vi "Parse MAVLink Message.vi"(11 "Instance Details":T2) -> ()   [LabVIEW 2014]
uses:
  Ground Station to Aircraft Coms/SubVI/Aircraft Data Router/Controls/Known Aircraft.ctl
  Ground Station to Aircraft Coms/SubVI/Hardware Driver/Controls/Coms Driver Interface.ctl
  Telemetry/Controls/Telemetry Connection Type.ctl
  <vilib>/httpClient/ClientHandle.ctl
  Controls/MAVLink Command ACK.ctl
  Aircraft Information/Controls/Drone Information.ctl
  Aircraft Information/Controls/Base Mode.ctl
  Aircraft Information/Controls/Aircraft Mode.ctl
  Aircraft Information/Controls/Aircraft Extra Data.ctl
  Controls/MAVLink Optical Flow.ctl
  Controls/MAVLink EKF Status Report.ctl
  Aircraft Information/Controls/Aircraft Sensor Status Data.ctl
  GUI Design/Indicators/Sensor Status LED CLuster.ctl
  GUI Design/Indicators/Status LED.ctl
  Aircraft Information/Controls/Aircraft GPS Data.ctl
  Aircraft Information/Controls/GPS Fix Type.ctl
  Aircraft Information/Controls/Aircraft Attitude Data.ctl
  Controls/MAVLink Recieved Param.ctl
  Aircraft Information/Sub VI/Set Aircraft System Status.vi
  Aircraft Information/Sub VI/Set Aircraft Information.vi
  Aircraft Information/Sub VI/Set Aircraft Extra Data.vi
  Aircraft Information/Sub VI/Set Aircraft GPS.vi
  Aircraft Information/Sub VI/Set Aircraft Attitude.vi
  Application Support/Stop Button/SubVI/Get Stop Button Status.vi
  <vilib>/httpClient/LabVIEWHTTPClient.lvlib
panel:
  out "output cluster":T1
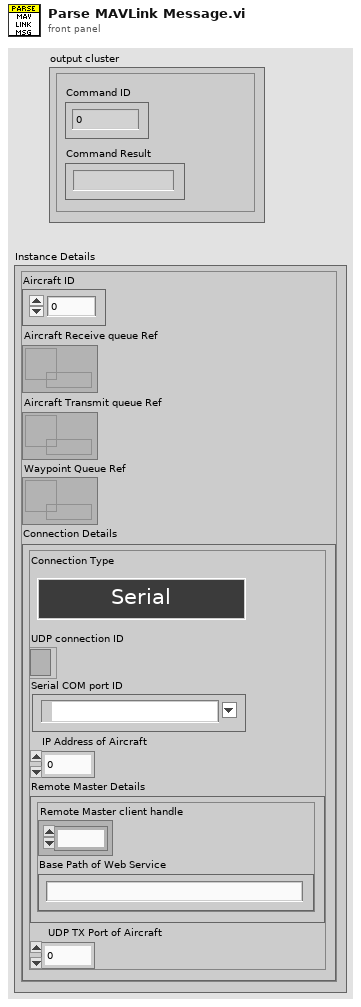
[diagram p1: front panel]
types:
  T1 = typedef "MAVLink Command ACK.ctl" = cluster{"Command ID":u16, "Command Result":string}
  T2 = typedef "Known Aircraft.ctl" = cluster{"Aircraft ID":u8, "Aircraft Receive queue Ref":refnum<queue>, "Aircraft Transmit queue Ref":refnum<queue>, "Waypoint Queue Ref":refnum<queue>, "Connection Details":T3}
  T3 = typedef "Coms Driver Interface.ctl" = cluster{"Connection Type":T4, "UDP connection ID":refnum<k16>, "Serial COM port ID":refnum<visa-resource-name>, "IP Address of Aircraft":u32, "Remote Master Details":cluster{"Remote Master client handle":T5, "Base Path of Web Service":string}, "UDP TX Port of Aircraft":u16}
  T4 = typedef "Telemetry Connection Type.ctl" = enum16{"Serial", "UDP", "Remote Master"}
  T5 = typedef "LabVIEWHTTPClient.lvlib/ClientHandle.ctl" = refnum<k1>
  T6 = typedef "Aircraft Attitude Data.ctl" = cluster{"Roll":sgl, "Pitch":sgl, "Yaw":sgl, "Timestamp":u32, "Update Frequency":dbl, "Altitude":sgl}
  T7 = typedef "Aircraft GPS Data.ctl" = cluster{"Latitude (degrees)":dbl, "Longitude (degrees)":dbl, "Altitude (m)":dbl, "Fix Type":T8, "HDOP (cm)":u16, "VDOP (cm)":u16, "Ground Speed (m/s)":dbl, "Coarse Over Ground (degrees)":u16, "Number of Satellites":u8}
  T8 = typedef "GPS Fix Type.ctl" = enum16{"No Fix 0", "No Fix 1", "2D Fix", "3D Fix", "DGPS", "RTK"}
  T9 = typedef "Aircraft Sensor Status Data.ctl" = cluster{"Sensor Status":T10, "CPU Load (%)":dbl, "Battery Voltage (V)":dbl, "Battery Current (A)":dbl, "Battery Remaining (%)":dbl, "Communication Drop Rate (%)":dbl, "Communication Errors (%)":dbl, "Status text":string}
  T10 = typedef "Sensor Status LED CLuster.ctl" = cluster{"3D Gyro":u32, "3D Accel":u32, "3D Mag":u32, "Abs. Pressure":u32, "Diff. Pressure":u32, "GPS":T11, "Optical Flow":u32, "Vision Position":u32, "Laser Position":u32, "External Ground Truth":u32, "Angular Rate Control":u32, "Attitude Stabilisation":u32, "Yaw Position":u32, "Z Altitude Control":u32, "XY Position Control":u32, "Motor Outputs":u32, "RC Receiver":u32, "3D Gyro 2":u32, "3D Accel 2":u32, "3D Mag 2":u32, "Geofence":u32, "AHRS":u32, "Terrain":u32}
  T11 = typedef "Status LED.ctl" = u32
  T12 = typedef "Aircraft Extra Data.ctl" = cluster{"Optical Flow":T13, "RNGFND Distance (m)":sgl, "RNGFND Voltage":sgl, "EKF Status Report":T14}
  T13 = typedef "MAVLink Optical Flow.ctl" = cluster{"Time (usec)":u64, "Flow Comp mx":sgl, "Flow Comp my":sgl, "Ground Distance (m)":sgl, "Flow x":i16, "Flow y":i16, "Sensord ID":u8, "Quality":u8}
  T14 = typedef "MAVLink EKF Status Report.ctl" = cluster{"EKF Status Flags":cluster{"Attitude Estimate":bool, "Horizontal Velocity":bool, "Vertical Velocity":bool, "Horizontal POS Relative":bool, "Horizontal POS Absolute":bool, "Vertical POS Relative":bool, "Vertical POS Absolute":bool, "Vertical POS AGL":bool, "Contstant POS Mode":bool, "Predicted Horizontal POS Relative":bool, "Predicted Horizontal POS Absolute":bool}, "Velocity Variance":sgl, "Horizontal POS Variance":sgl, "Vertical POS Variance":sgl, "Compass Variance":sgl, "Terrain Altitude Variance":sgl}
  T15 = typedef "Drone Information.ctl" = cluster{"Aircraft ID":u8, "Tag ID":string, "System Status":string, "Base Mode":T16, "Armed/Disarmed":bool, "Battery Voltage":dbl, "Control Mode":T17, "Initialisation":u8, "Coms with aircraft good":bool, "Mode":string, "Mission Uploaded":bool}
  T16 = typedef "Base Mode.ctl" = cluster{"Custom Mode":bool, "Test Enabled":bool, "Autonomous Mode":bool, "Guided Mode":bool, "Stabilization Enabled":bool, "HIL Enabled":bool, "Manual Mode":bool, "Arm":bool}
  T17 = typedef "Aircraft Mode.ctl" = enum16{"Loiter", "Stabalise", "Failsafe", "Emergency Stop"}
  T18 = typedef "MAVLink Recieved Param.ctl" = cluster{"Param ID":string, "Param Value":sgl, "Param Type":u8, "Param Count":u16, "Param Index":u16}
  T19 = enum16{"ALL", "RAW_SENSORS", "EXTENDED_STATUS", "RC_CHANNELS", "RAW_CONTROLLER", "POSITION", "EXTRA1", "EXTRA2", "EXTRA3"}
  T20 = cluster{"x acc":i16, "y acc":i16, "z acc":i16, "x gyro":i16, "y gyro":i16, "z gyro":i16, "x mag":i16, "y mag":i16, "z mag":i16}
  T21 = cluster{"Channel 1":u16, "Channel 2":u16, "Channel 3":u16, "Channel 4":u16, "Channel 5":u16, "Channel 6":u16, "Channel 7":u16, "Channel 8":u16}
  T22 = typedef "MAVLink Packet.ctl" = cluster{"Payload Length":u8, "Packet Sequence":u8, "System ID":u8, "Component ID":u8, "Message ID":u8, "Data":string, "Checksum":u16}
  T23 = typedef "MAVLink Heartbeat.ctl" = cluster{"custom_mode":u32, "Type":u8, "autopilot":u8, "base_mode":u8, "system_status":u8, "mavlink_version":u8, "heartbeat":bool}
  T24 = typedef "MAVLink System Status.ctl" = cluster{"onboard_control_sesnors_present":u32, "onboard_control_sesnors_enabled":u32, "onboard_control_sesnors_health":u32, "load (%*10)":u16, "voltage_battery (mV)":u16, "current_battery (mA*10)":i16, "drop_rate_comm (%*100)":u16, "error_comm":u16, "error_count1":u16, "error_count2":u16, "error_count3":u16, "error_count4":u16, "battery_remaining (%)":i8}
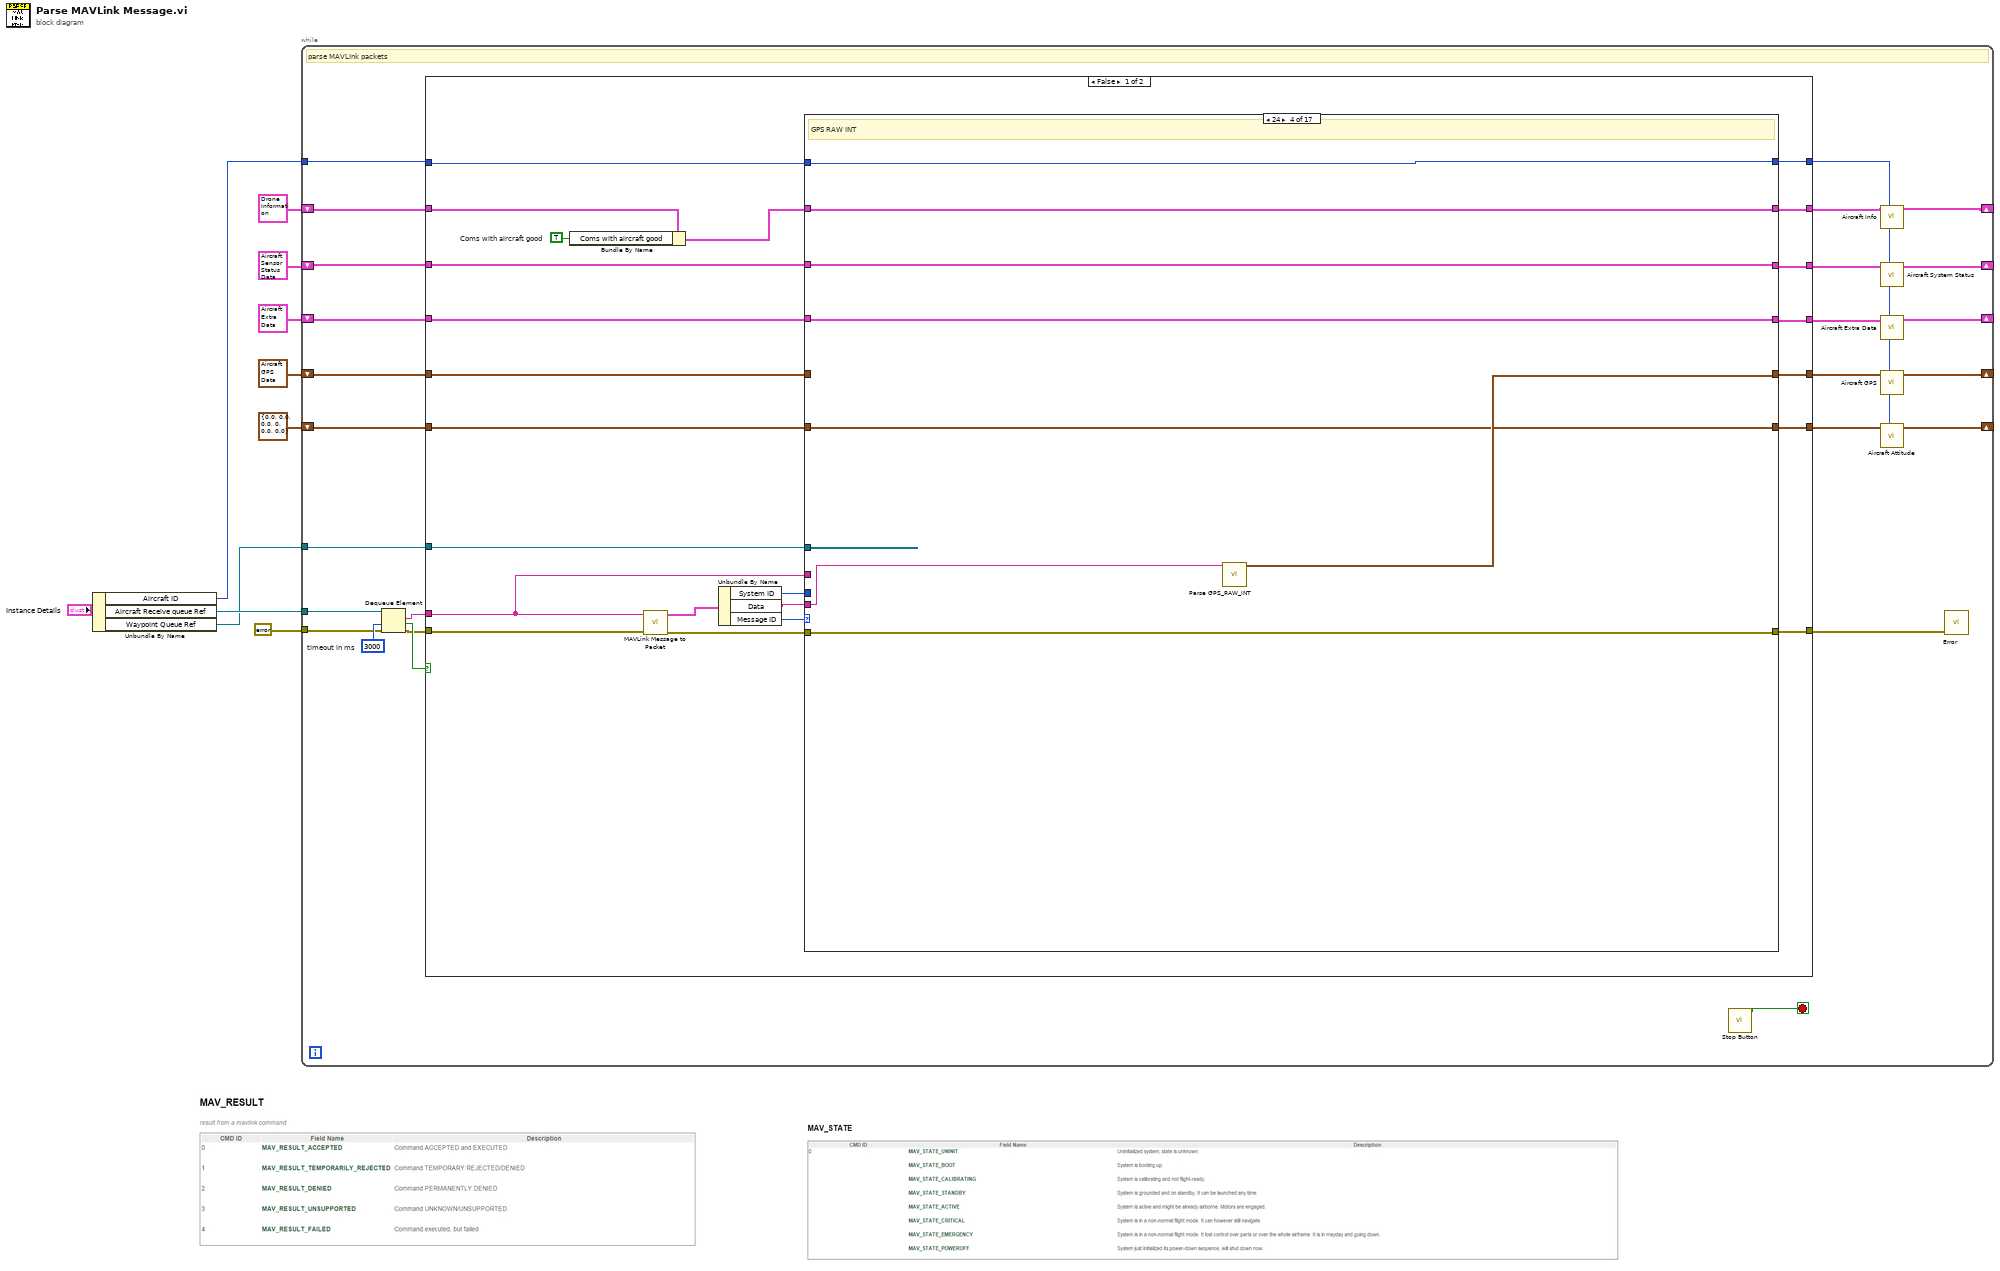
[diagram p0: block diagram]
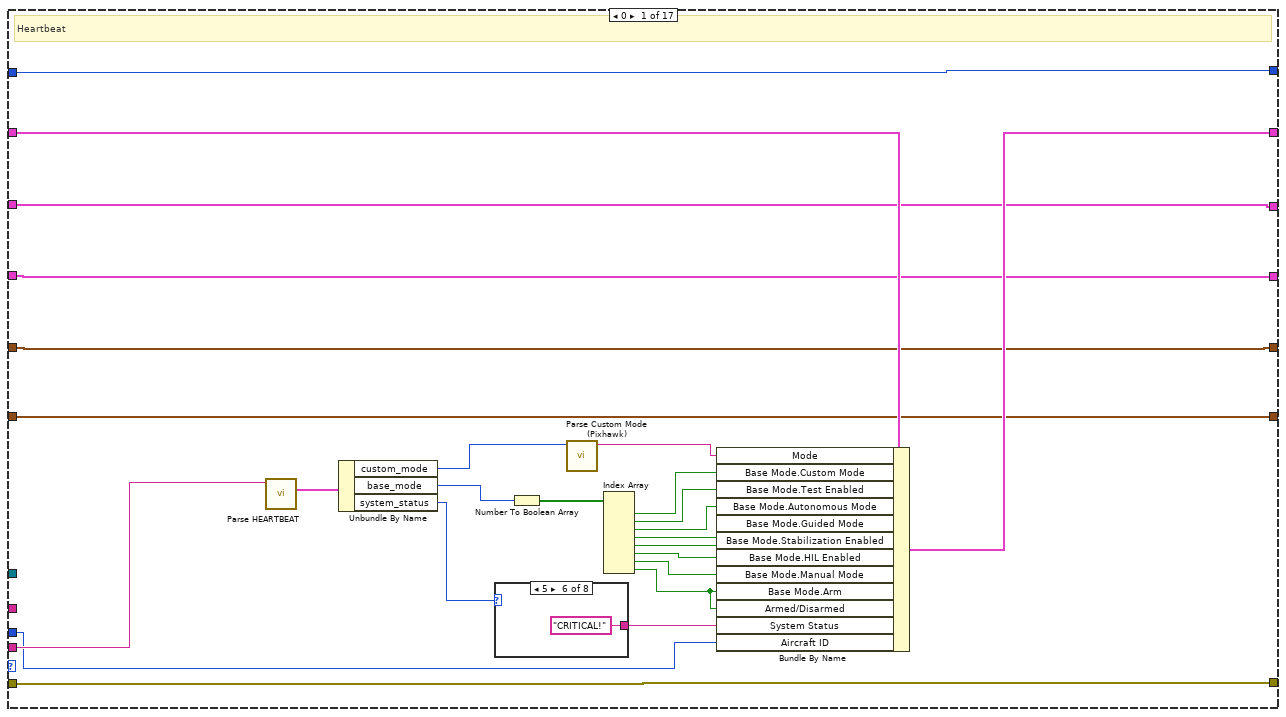
[diagram p2: hidden frame]
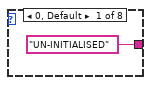
[diagram p3: hidden frame]
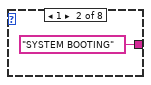
[diagram p4: hidden frame]
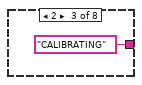
[diagram p5: hidden frame]
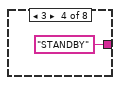
[diagram p6: hidden frame]
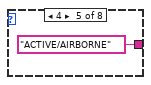
[diagram p7: hidden frame]
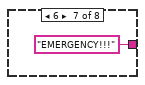
[diagram p8: hidden frame]
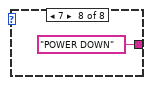
[diagram p9: hidden frame]
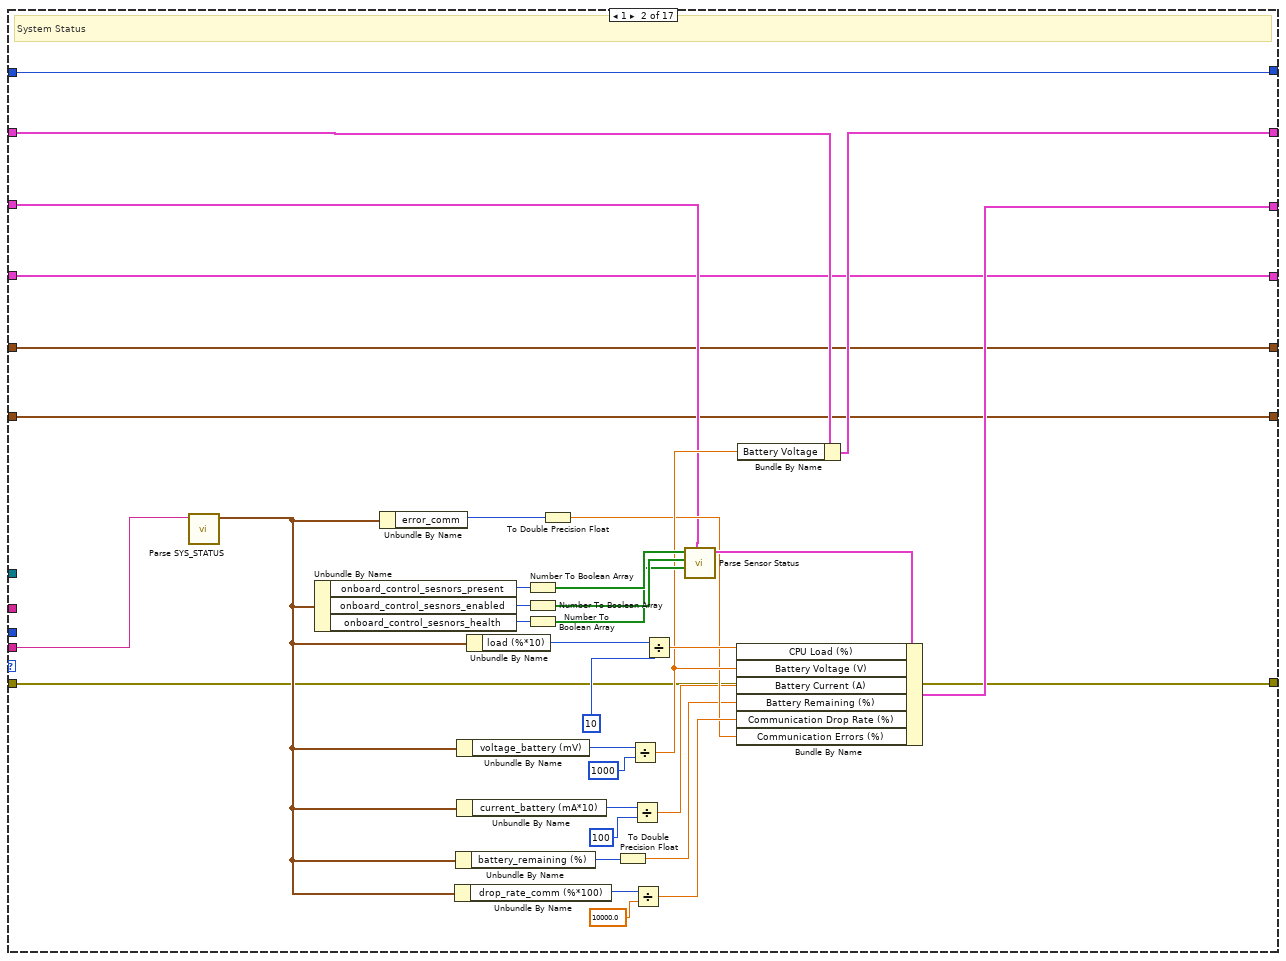
[diagram p10: hidden frame]
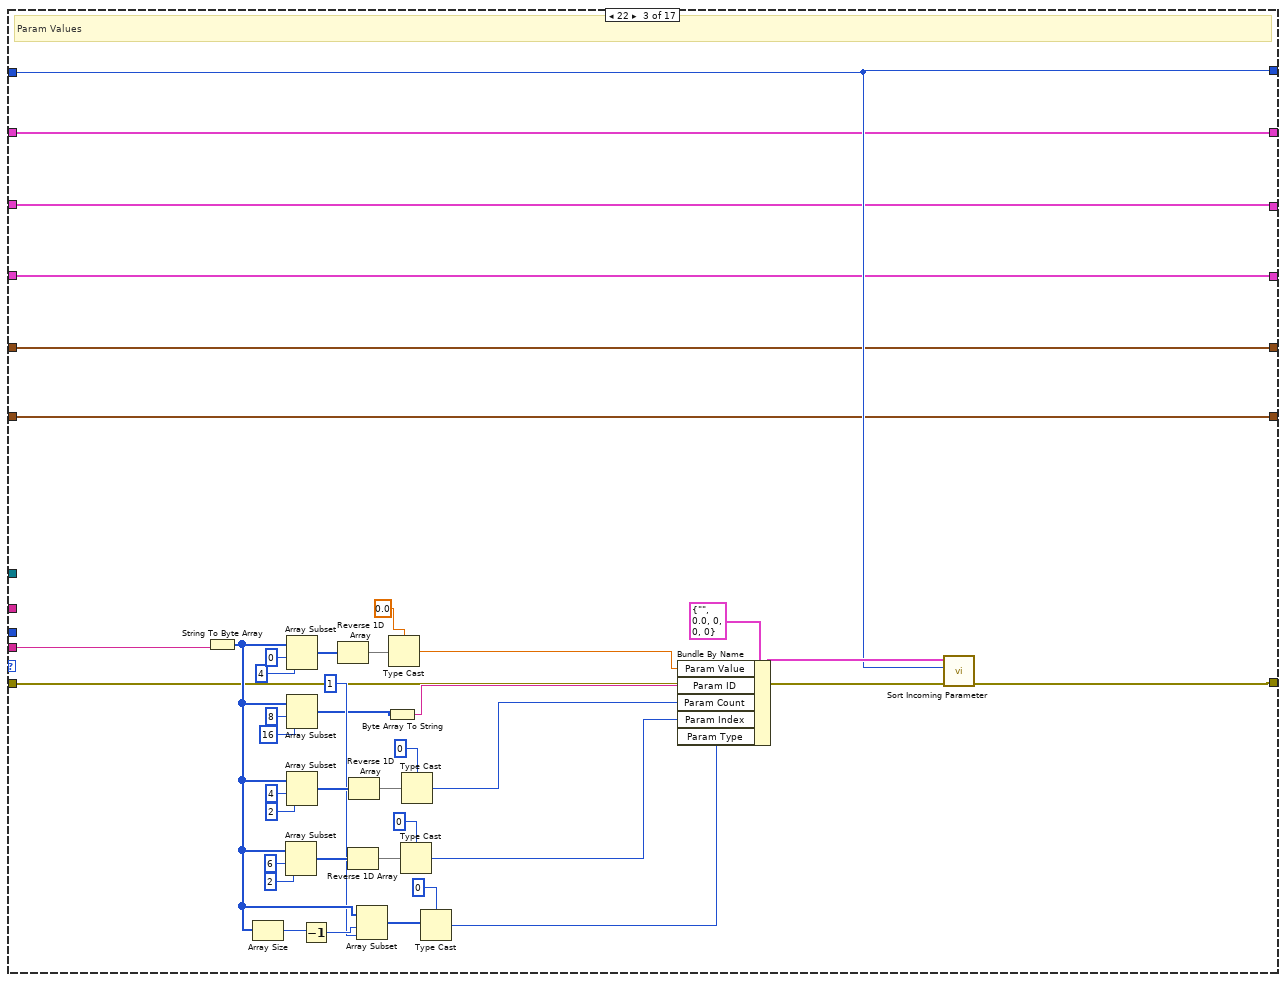
[diagram p11: hidden frame]
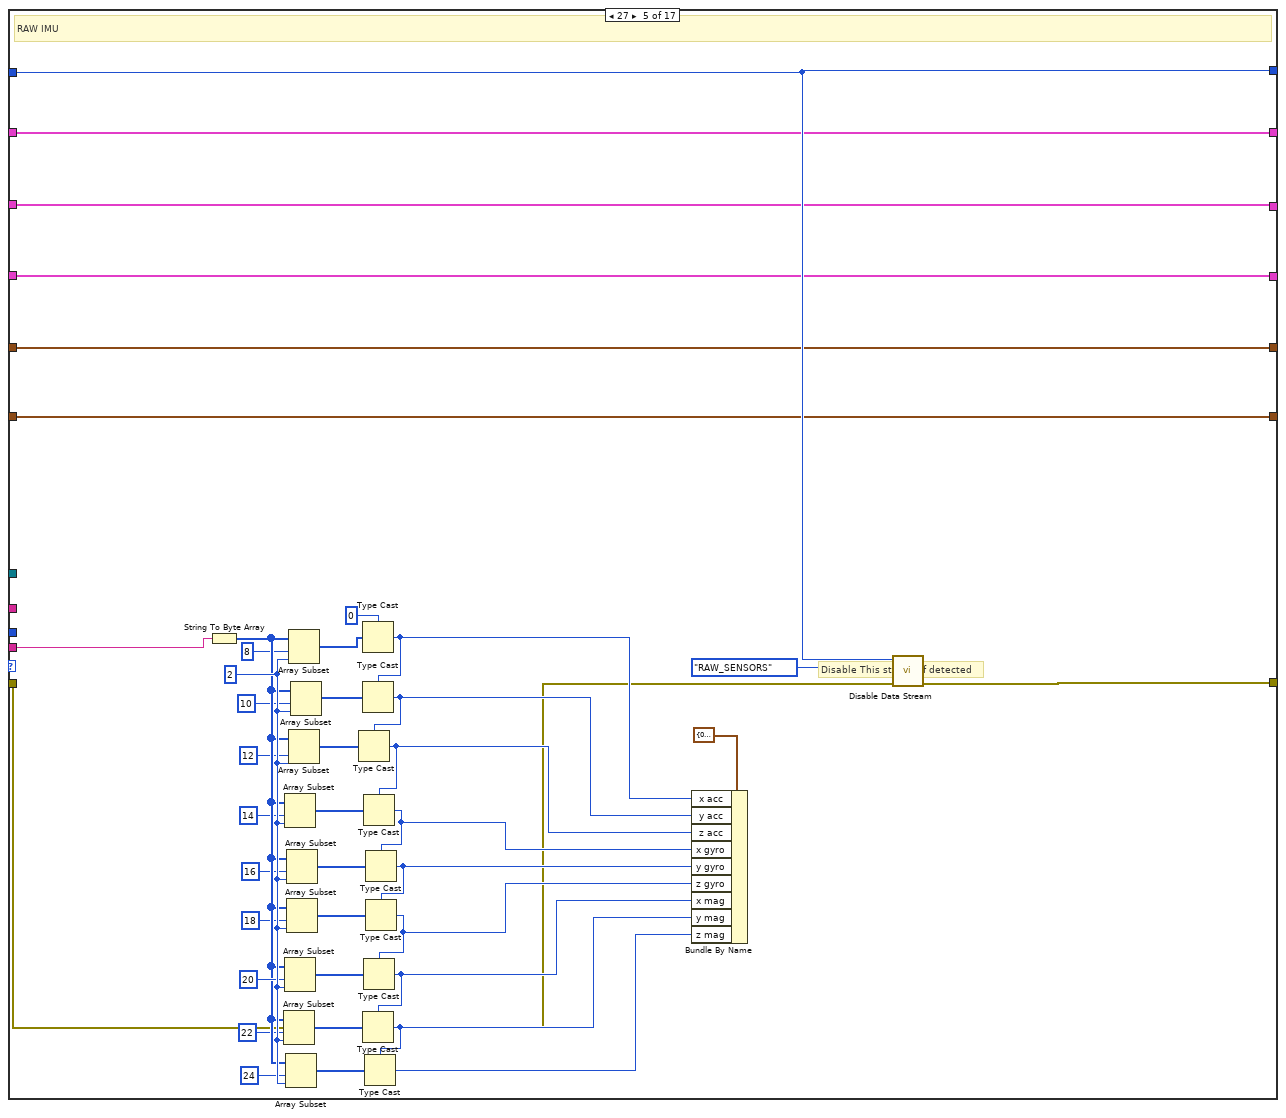
[diagram p12: hidden frame]
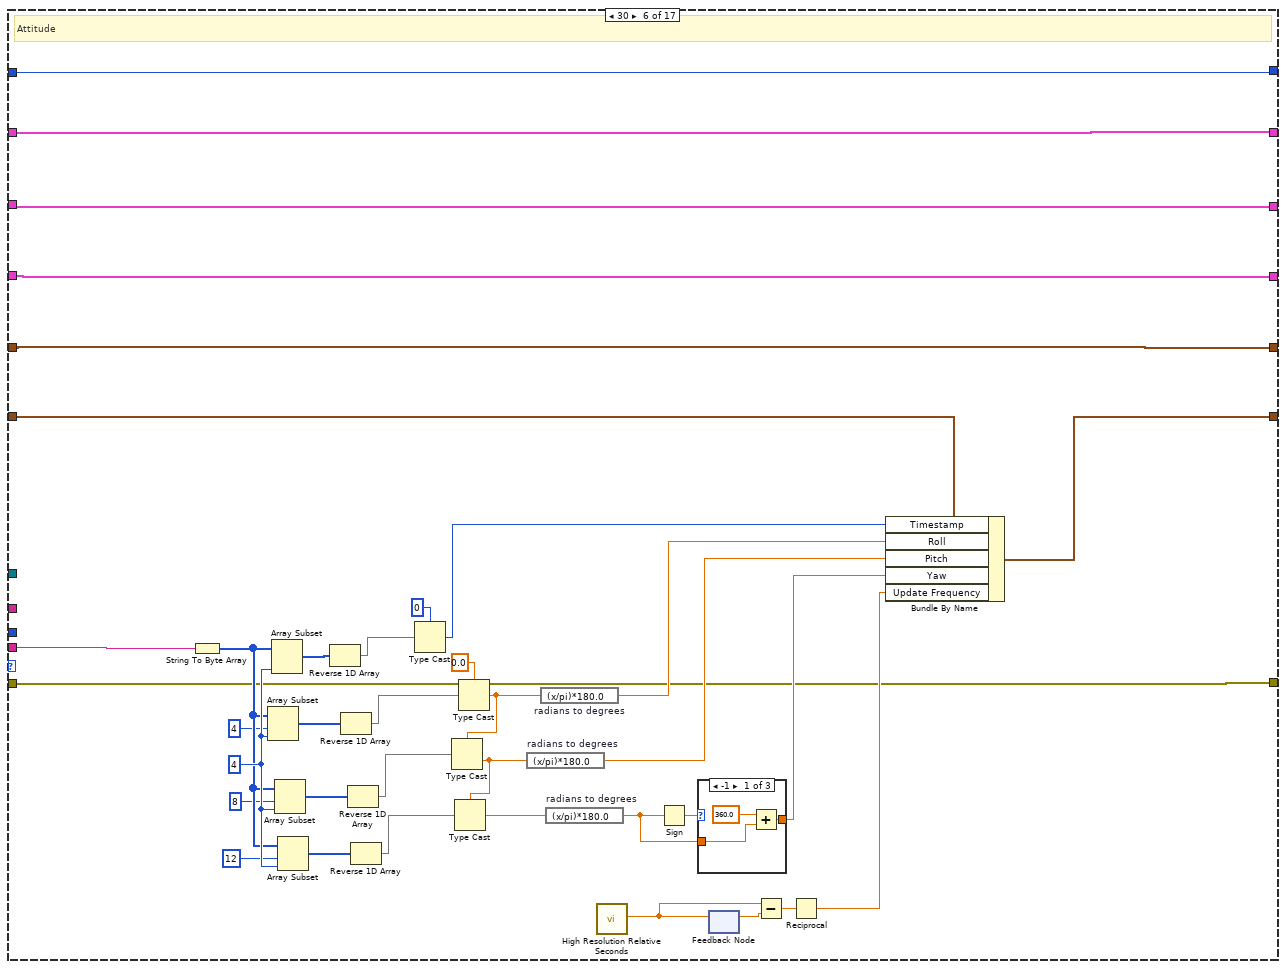
[diagram p13: hidden frame]
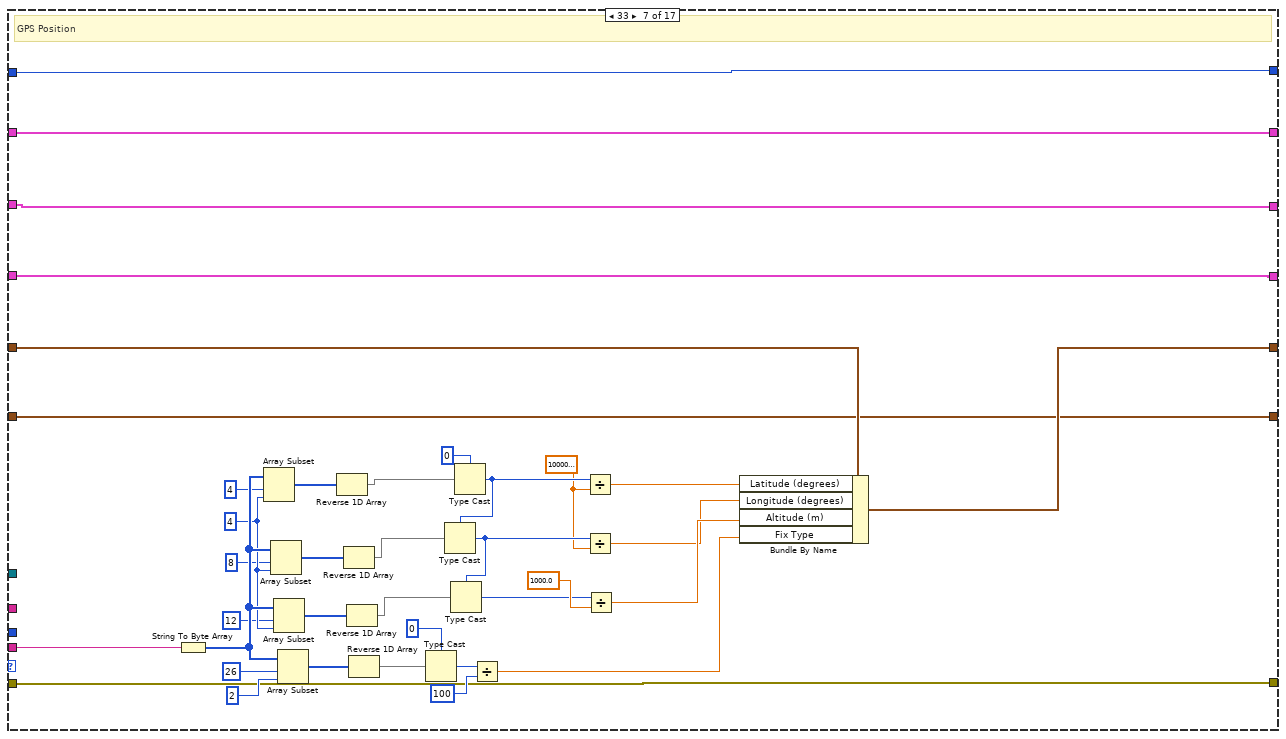
[diagram p16: hidden frame]
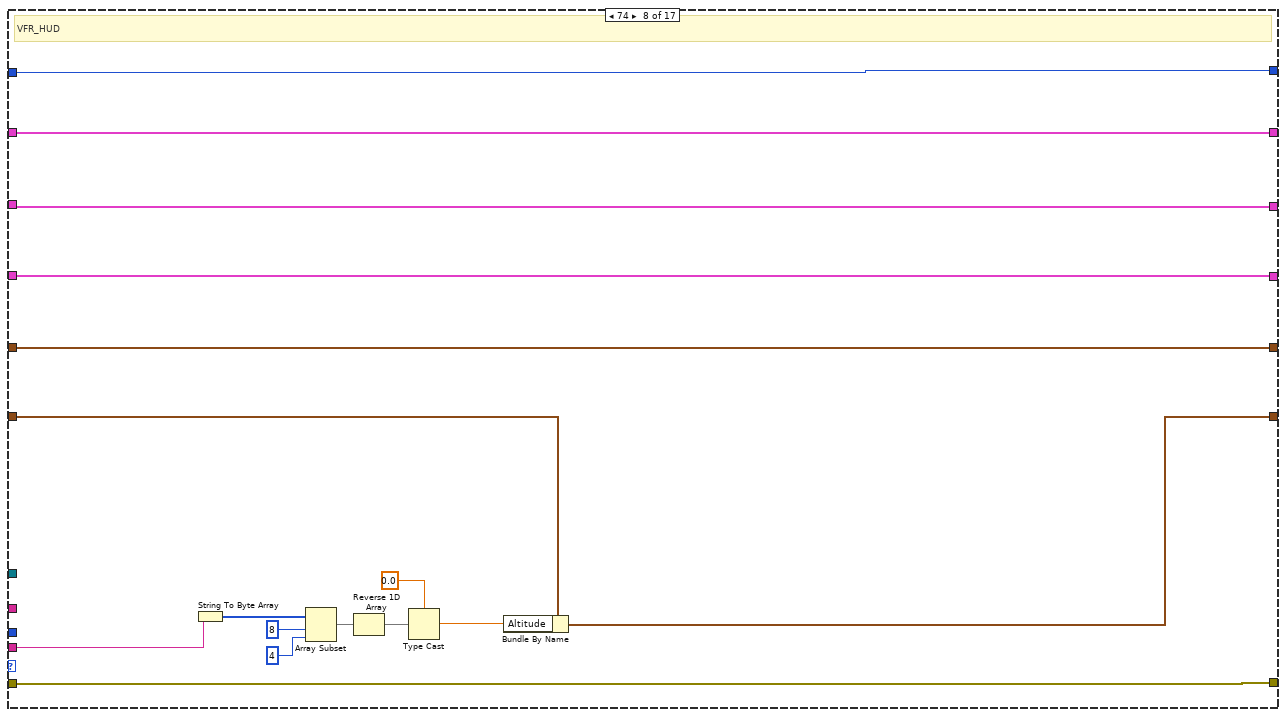
[diagram p17: hidden frame]
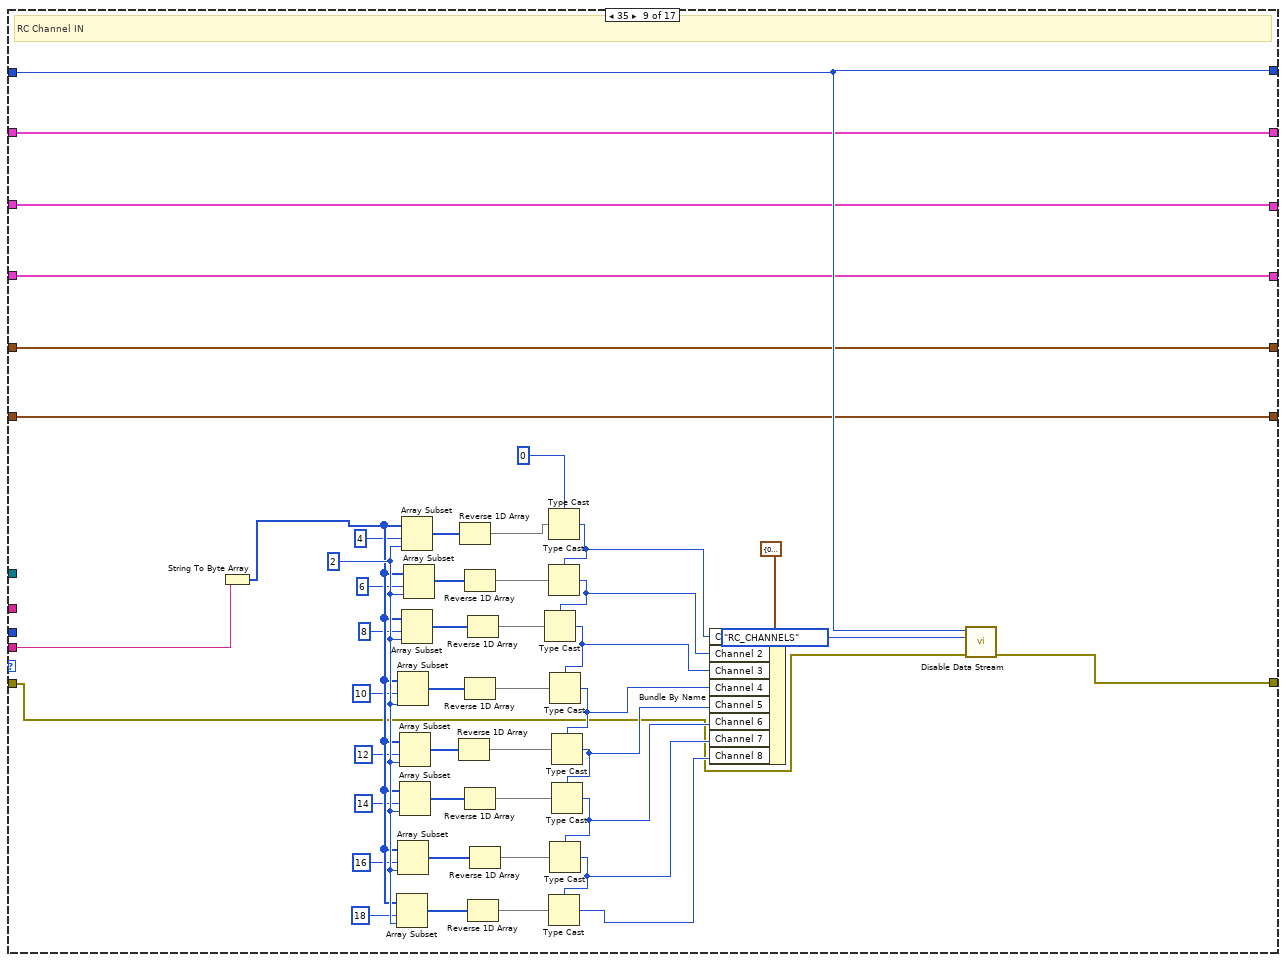
[diagram p18: hidden frame]
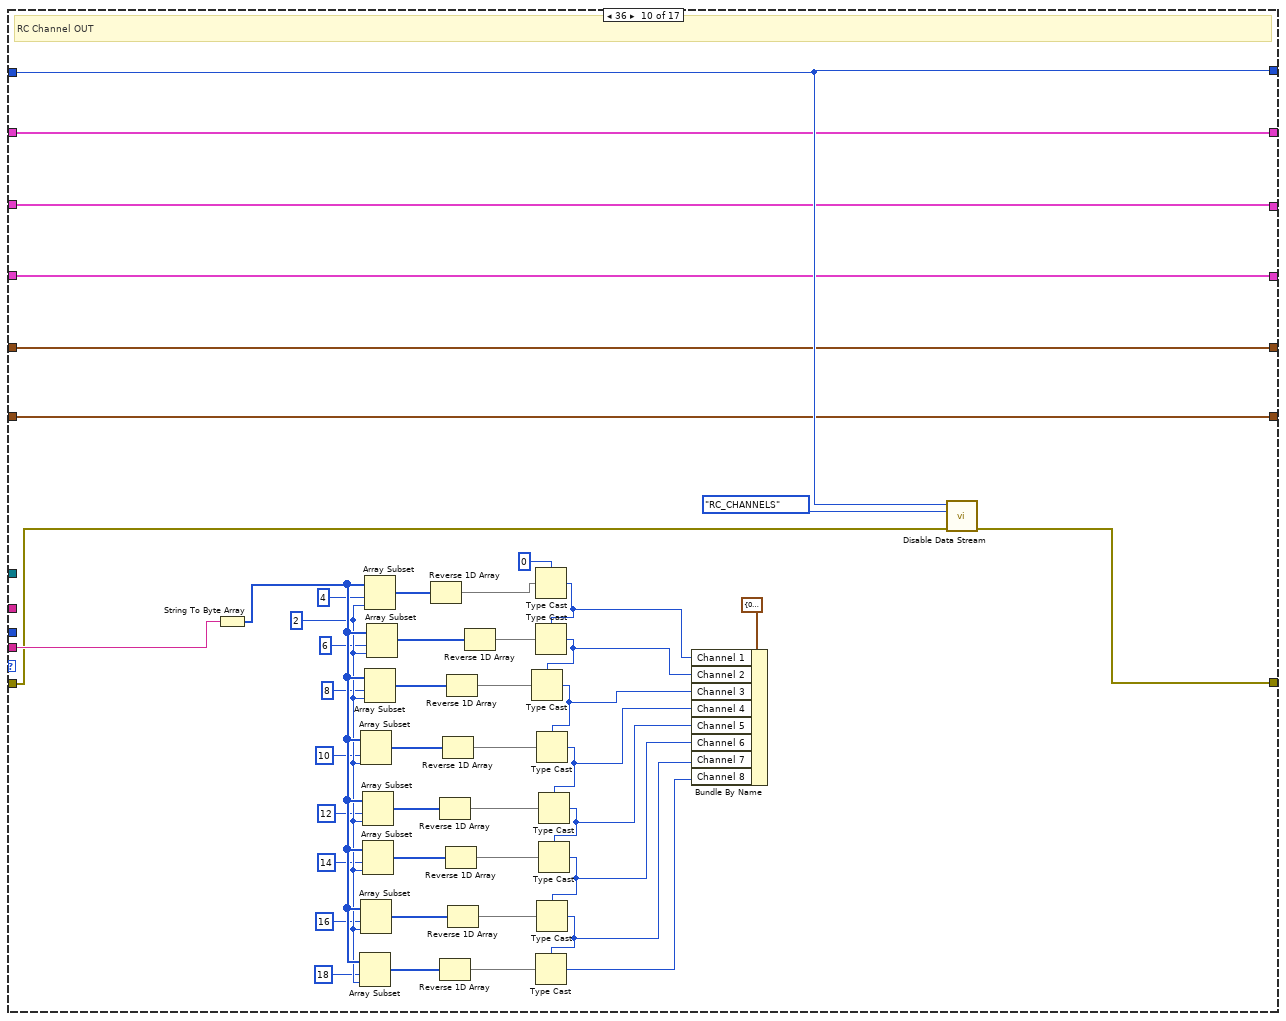
[diagram p19: hidden frame]
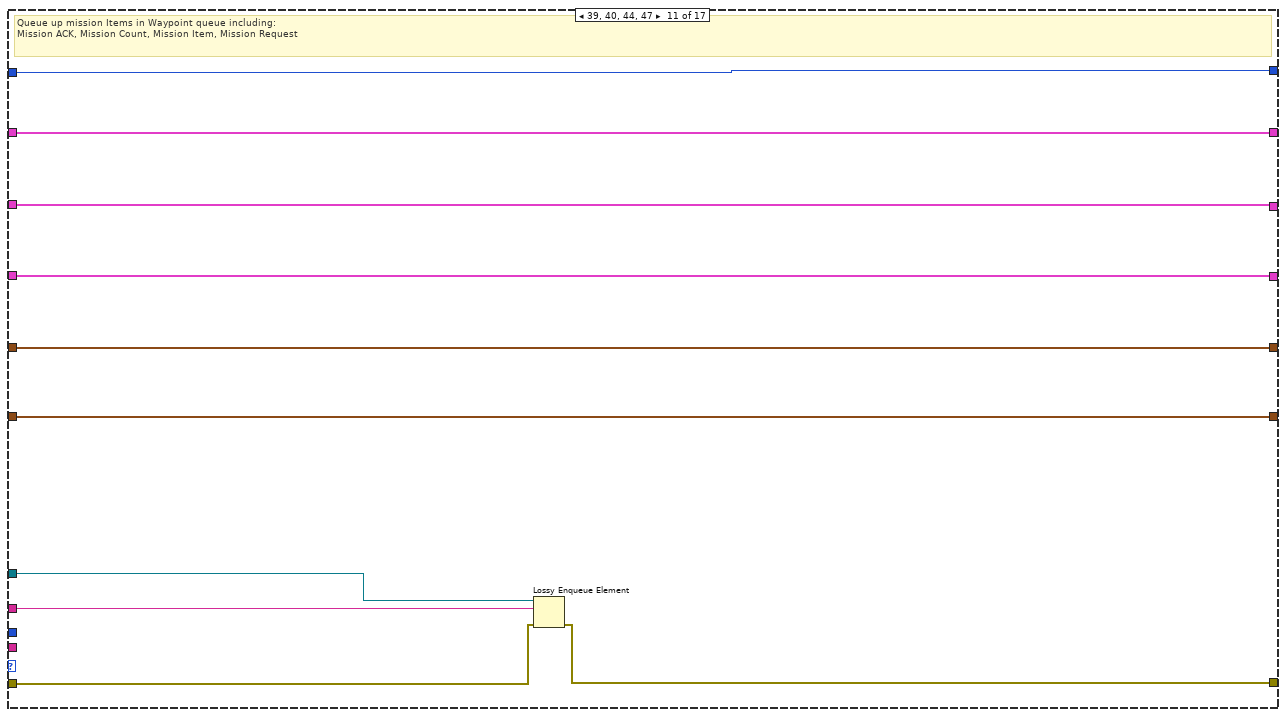
[diagram p20: hidden frame]
diagram:
  n1 = Unbundle By Name("Instance Details") -> ("Aircraft ID"=w8:u8, "Aircraft Receive queue Ref"=w7:refnum<queue>, "Waypoint Queue Ref"=w6:refnum<queue>)
  n2 = while {
    tunnel: w8 -> [w31]
    tunnel: w7 -> [w30]
    tunnel: w6 -> [w29]
    tunnel: errorcluster {"status"=FALSE, "code"=0, "source"=""} ("error in (no error)") -> [w32]
    shift-right: [w23] -> _
    shift-left: T15 {"Aircraft ID"=0, "Tag ID"="", "System Status"="", "Base Mode"={"Custom Mode"=FALSE, "Test Enabled"=FALSE, "Autonomous Mode"=FALSE, "Guided Mode"=FALSE, "Stabilization Enabled"=FALSE, "HIL Enabled"=FALSE, "Manual Mode"=FALSE, "Arm"=FALSE}, "Armed/Disarmed"=FALSE, "Battery Voltage"=0.0, "Control Mode"=enum."Stabalise", "Initialisation"=0, "Coms with aircraft good"=FALSE, "Mode"="", "Mission Uploaded"=FALSE} ("Aircraft Information Out") -> [w26]
    shift-right: [w25] -> _
    shift-left: T9 {"Sensor Status"={"3D Gyro"=0, "3D Accel"=0, "3D Mag"=0, "Abs. Pressure"=0, "Diff. Pressure"=0, "GPS"=0, "Optical Flow"=0, "Vision Position"=0, "Laser Position"=0, "External Ground Truth"=0, "Angular Rate Control"=0, "Attitude Stabilisation"=0, "Yaw Position"=0, "Z Altitude Control"=0, "XY Position Control"=0, "Motor Outputs"=0, "RC Receiver"=0, "3D Gyro 2"=0, "3D Accel 2"=0, "3D Mag 2"=0, "Geofence"=0, "AHRS"=0, "Terrain"=0}, "CPU Load (%)"=0.0, "Battery Voltage (V)"=0.0, "Battery Current (A)"=0.0, "Battery Remaining (%)"=0.0, "Communication Drop Rate (%)"=0.0, "Communication Errors (%)"=0.0, "Status text"=""} ("System Status Out") -> [w24]
    shift-right: [w19] -> _
    shift-left: T12 {"Optical Flow"={"Time (usec)"=0, "Flow Comp mx"=0.0, "Flow Comp my"=0.0, "Ground Distance (m)"=0.0, "Flow x"=0, "Flow y"=0, "Sensord ID"=0, "Quality"=0}, "RNGFND Distance (m)"=0.0, "RNGFND Voltage"=0.0, "EKF Status Report"={"EKF Status Flags"={"Attitude Estimate"=FALSE, "Horizontal Velocity"=FALSE, "Vertical Velocity"=FALSE, "Horizontal POS Relative"=FALSE, "Horizontal POS Absolute"=FALSE, "Vertical POS Relative"=FALSE, "Vertical POS Absolute"=FALSE, "Vertical POS AGL"=FALSE, "Contstant POS Mode"=FALSE, "Predicted Horizontal POS Relative"=FALSE, "Predicted Horizontal POS Absolute"=FALSE}, "Velocity Variance"=0.0, "Horizontal POS Variance"=0.0, "Vertical POS Variance"=0.0, "Compass Variance"=0.0, "Terrain Altitude Variance"=0.0}} ("Extra Data Out") -> [w20]
    shift-right: [w17] -> _
    shift-left: T7 {"Latitude (degrees)"=0.0, "Longitude (degrees)"=0.0, "Altitude (m)"=0.0, "Fix Type"=enum."No Fix 0", "HDOP (cm)"=0, "VDOP (cm)"=0, "Ground Speed (m/s)"=0.0, "Coarse Over Ground (degrees)"=0, "Number of Satellites"=0} ("Aircraft Att Data Out") -> [w16]
    shift-right: [w13] -> _
    shift-left: T6 {"Roll"=0.0, "Pitch"=0.0, "Yaw"=0.0, "Timestamp"=0, "Update Frequency"=0.0, "Altitude"=0.0} ("Aircraft Att Data Out") -> [w12]
    stop <- w28 stop-if-true
    w36 = 3000  # timeout in ms
    # "parse MAVLink packets"
    n3 = Dequeue Element(queue=w30, timeout in ms (-1)=w36, error in (no error)=w32) -> (element=w33:string, timed out?=w35:bool, error out=w34:errorcluster)  [unwired: 1 out]
    n4 = case shown="False" w35 {
      tunnel: w34 -> [w40 w512]
      tunnel: [w57 w512] -> w27
      tunnel: w31 -> [w54 w507]
      tunnel: w33 -> [w41 _]
      tunnel: w29 -> [w55 _]
      tunnel: w26 -> [w38 w506]
      tunnel: [w53 w507] -> w14
      tunnel: w24 -> [w50 w511]
      tunnel: [w51 w505] -> w22
      tunnel: [w49 w511] -> w21
      tunnel: w20 -> [w47 w510]
      tunnel: [w46 w510] -> w18
      tunnel: w16 -> [w45 w509]
      tunnel: [w44 w509] -> w15
      tunnel: w12 -> [w42 w508]
      tunnel: [w43 w508] -> w11
      frame False {
        w39 = TRUE  # Coms with aircraft good
        n5 = Bundle By Name(cluster=w38, "Coms with aircraft good"=w39) -> (w37:T15)
        n6 = call "MAVLink Message to Packet.vi"("Error In"=w40, "Message"=w41) -> ("Error Out"=w52:errorcluster, "Packet"=w56:T22)  [unwired: 8 in]
        n7 = Unbundle By Name(w56) -> ("System ID"=w48:u8, "Data"=w58:string, "Message ID"=w59:u8)
        n8 = case shown="24" w59 {
          tunnel: w58 -> [w73 w112 w166 w174 w185 w229 w266 w307 w320 w375 _ w436 w454 w465 w475 w496 _]
          tunnel: w48 -> [w64 _ _ _ _ _ _ _ _ _ _ _ _ _ _ _ _]
          tunnel: w52 -> [w65 w93 w134 w168 w182 w217 w265 w298 w318 w363 w410 w417 w449 w459 w471 w478 w503]
          tunnel: [w65 w93 w130 w168 w183 w217 w265 w298 w319 w364 w409 w417 w449 w459 w471 w478 w503] -> w57
          tunnel: w37 -> [w74 w113 w132 w172 w178 w216 w261 w297 w314 w360 w406 w419 w447 w458 w469 w479 w501]
          tunnel: w54 -> [w69 w100 w133 w173 w180 w223 w264 w302 w316 w362 w408 w421 w452 w462 w473 w483 w502]
          tunnel: w41 -> [_ _ _ _ _ _ _ _ _ _ w411 _ _ _ _ _ _]
          tunnel: w55 -> [_ _ _ _ _ _ _ _ _ _ w412 _ _ _ _ _ _]
          tunnel: [w69 w100 w133 w173 w180 w223 w264 w302 w316 w362 w408 w421 w452 w462 w473 w483 w502] -> w53
          tunnel: [w66 w99 w132 w172 w178 w216 w261 w297 w314 w360 w406 w419 w447 w458 w469 w479 w501] -> w51
          tunnel: w50 -> [w63 w98 w131 w171 w177 w219 w260 w296 w313 w359 w405 w420 w446 w457 w468 w482 w500]
          tunnel: [w63 w97 w131 w171 w177 w219 w260 w296 w313 w359 w405 w418 w446 w457 w468 w481 w500] -> w49
          tunnel: w47 -> [w62 w96 w129 w170 w176 w218 w259 w295 w312 w358 w404 w414 w451 w461 w472 w480 w499]
          tunnel: [w62 w96 w129 w170 w176 w218 w259 w295 w312 w358 w404 w414 w450 w460 w470 w480 w499] -> w46
          tunnel: w45 -> [w61 w95 w128 _ w179 w222 w263 w301 w315 w361 w407 w415 w448 w456 w467 w477 w498]
          tunnel: [w61 w95 w128 w169 w179 w222 w262 w301 w315 w361 w407 w415 w448 w456 w467 w477 w498] -> w44
          tunnel: [w60 w94 w127 w167 w175 w220 w258 w299 w311 w357 w403 w413 w445 w455 w466 w476 w497] -> w43
          tunnel: w42 -> [w60 w94 w127 w167 w175 w221 w258 w300 w311 w357 w403 w413 w445 w455 w466 w476 w497]
          frame 0 {
            # "Heartbeat"
            n9 = call "Parse HEARTBEAT.vi"("Data"=w73) -> ("Heartbeat"=w72:T23)  [unwired: 10 in]
            n10 = Unbundle By Name(w72) -> ("custom_mode"=w68:u32, "base_mode"=w70:u8, "system_status"=w71:u8)
            n11 = case shown="5" w71 {
              tunnel: ["UN-INITIALISED" "SYSTEM BOOTING" "CALIBRATING" "STANDBY" "ACTIVE/AIRBORNE" "CRITICAL!" "EMERGENCY!!!" "POWER DOWN"] -> w75
              frame 0, Default {
              }
              frame 1 {
              }
              frame 2 {
              }
              frame 3 {
              }
              frame 4 {
              }
              frame 5 {
              }
              frame 6 {
              }
              frame 7 {
              }
            }
            n12 = Number To Boolean Array(number=w70) -> (Boolean array=w84:bool[])
            n13 = call "Parse Custom Mode (Pixhawk).vi"("custom mode"=w68) -> ("Custom Mode"=w67:string)  [unwired: 9 in, 1 out]
            n14 = Index Array(array=w84) -> (element #1=w83:bool, element #2=w82:bool, element #3=w81:bool, element #4=w80:bool, element #5=w79:bool, element #6=w78:bool, element #7=w77:bool, element #8=w76:bool)  [unwired: 8 in]
            n15 = Bundle By Name(cluster=w74, "Mode"=w67, "Base Mode.Custom Mode"=w83, "Base Mode.Test Enabled"=w82, "Base Mode.Autonomous Mode"=w81, "Base Mode.Guided Mode"=w80, "Base Mode.Stabilization Enabled"=w79, "Base Mode.HIL Enabled"=w78, "Base Mode.Manual Mode"=w77, "Base Mode.Arm"=w76, "Armed/Disarmed"=w76, "System Status"=w75, "Aircraft ID"=w64) -> (w66:T15)
          }
          frame 1 {
            # "System Status"
            n16 = call "Parse SYS_STATUS.vi"("Data"=w112) -> ("System Status"=w102:T24)  [unwired: 10 in]
            n17 = Unbundle By Name(w102) -> ("onboard_control_sesnors_present"=w111:u32, "onboard_control_sesnors_enabled"=w110:u32, "onboard_control_sesnors_health"=w109:u32)
            n18 = Unbundle By Name(w102) -> ("error_comm"=w101:u16)
            n19 = Unbundle By Name(w102) -> ("drop_rate_comm (%*100)"=w103:u16)
            n20 = Unbundle By Name(w102) -> ("battery_remaining (%)"=w105:i8)
            n21 = Unbundle By Name(w102) -> ("voltage_battery (mV)"=w107:u16)
            n22 = Unbundle By Name(w102) -> ("current_battery (mA*10)"=w106:i16)
            n23 = Unbundle By Name(w102) -> ("load (%*10)"=w108:u16)
            n24 = Number To Boolean Array(number=w111) -> (Boolean array=w124:bool[])
            n25 = Number To Boolean Array(number=w110) -> (Boolean array=w123:bool[])
            n26 = Number To Boolean Array(number=w109) -> (Boolean array=w122:bool[])
            n27 = To Double Precision Float(number=w101) -> (double precision float=w115:dbl)
            n28 = To Double Precision Float(number=w105) -> (double precision float=w104:dbl)
            n29 = Divide(x=w107, y=u16 1000) -> (x/y=w118:dbl)
            n30 = Divide(x=w106, y=i16 100) -> (x/y=w114:dbl)
            n31 = Divide(x=w103, y=10000.0) -> (x/y=w116:dbl)
            n32 = Divide(x=w108, y=u16 10) -> (x/y=w119:dbl)
            n33 = call "Parse Sensor Status.vi"("Aircraft System Status"=w98, "Healthy"=w122, "Enabled"=w123, "Present"=w124) -> ("Aircraft System Status Out"=w121:T9)  [unwired: 7 in]
            n34 = Bundle By Name(cluster=w121, "CPU Load (%)"=w119, "Battery Voltage (V)"=w118, "Battery Current (A)"=w114, "Battery Remaining (%)"=w104, "Communication Drop Rate (%)"=w116, "Communication Errors (%)"=w115) -> (w97:T9)
            n35 = Bundle By Name(cluster=w113, "Battery Voltage"=w118) -> (w99:T15)
          }
          frame 22 {
            # "Param Values"
            n36 = String To Byte Array(string=w166) -> (unsigned byte array=w145:u8[])
            n37 = Array Size(array=w145) -> (size(s)=w146:i32)
            n38 = Array Subset(array=w145, index=6, length=2) -> (w151:u8[])
            n39 = Array Subset(array=w145, index=0, length=4) -> (w163:u8[])
            n40 = Array Subset(array=w145, index=8, length=16) -> (w137:u8[])
            n41 = Array Subset(array=w145, index=4, length=2) -> (w156:u8[])
            n42 = Decrement(x=w146) -> (x-1=w144:i32)
            n43 = Reverse 1D Array(array=w163) -> (reversed array=w162:u8[])
            n44 = Reverse 1D Array(array=w151) -> (reversed array=w152:u8[])
            n45 = Reverse 1D Array(array=w156) -> (reversed array=w155:u8[])
            n46 = Array Subset(array=w145, index=w144, length=1) -> (w142:u8[])
            n47 = Byte Array To String(unsigned byte array=w137) -> (string=w139:string)
            n48 = Type Cast(type=sgl 0.0, x=w162) -> (*(type *) &x=w138:sgl)
            n49 = Type Cast(type=u16 0, x=w152) -> (*(type *) &x=w147:u16)
            n50 = Type Cast(type=u16 0, x=w155) -> (*(type *) &x=w153:u16)
            n51 = Type Cast(type=u8 0, x=w142) -> (*(type *) &x=w140:u8)
            n52 = Bundle By Name(cluster=T18 {"Param ID"="", "Param Value"=0.0, "Param Type"=0, "Param Count"=0, "Param Index"=0} ("Param Value Out"), "Param Value"=w138, "Param ID"=w139, "Param Count"=w153, "Param Index"=w147, "Param Type"=w140) -> (w136:T18)
            n53 = call "Sort Incoming Parameter.vi"("Error In"=w134, "Aircraft ID"=w133, "Param Value"=w136) -> ("Error Out"=w130:errorcluster)  [unwired: 8 in]
          }
          frame 24 {
            # "GPS RAW INT"
            n54 = call "Parse GPS_RAW_INT.vi"("Data"=w174) -> ("GPS Data Out"=w169:T7)  [unwired: 10 in]
          }
          frame 27 {
            w206 = 2 ("length")
            # "Disable This stream if detected"
            # "RAW IMU"
            n55 = String To Byte Array(string=w185) -> (unsigned byte array=w204:u8[])
            n56 = Array Subset(array=w204, index=22, length=w206) -> (w199:u8[])
            n57 = Array Subset(array=w204, index=14, length=w206) -> (w188:u8[])
            n58 = Array Subset(array=w204, index=20, length=w206) -> (w203:u8[])
            n59 = Array Subset(array=w204, index=24, length=w206) -> (w202:u8[])
            n60 = Array Subset(array=w204, index=16, length=w206) -> (w195:u8[])
            n61 = Array Subset(array=w204, index=18, length=w206) -> (w198:u8[])
            n62 = Array Subset(array=w204, index=8, length=w206) -> (w193:u8[])
            n63 = Array Subset(array=w204, index=12, length=w206) -> (w187:u8[])
            n64 = Array Subset(array=w204, index=10, length=w206) -> (w194:u8[])
            n65 = Type Cast(type=i16 0, x=w193) -> (*(type *) &x=w207:i16)
            n66 = Type Cast(type=w207, x=w194) -> (*(type *) &x=w208:i16)
            n67 = Type Cast(type=w208, x=w187) -> (*(type *) &x=w209:i16)
            n68 = Type Cast(type=w209, x=w188) -> (*(type *) &x=w215:i16)
            n69 = Type Cast(type=w215, x=w195) -> (*(type *) &x=w210:i16)
            n70 = Type Cast(type=w210, x=w198) -> (*(type *) &x=w211:i16)
            n71 = Type Cast(type=w211, x=w203) -> (*(type *) &x=w212:i16)
            n72 = Type Cast(type=w212, x=w199) -> (*(type *) &x=w213:i16)
            n73 = Type Cast(type=w213, x=w202) -> (*(type *) &x=w214:i16)
            n74 = Bundle By Name(cluster=T20 {"x acc"=0, "y acc"=0, "z acc"=0, "x gyro"=0, "y gyro"=0, "z gyro"=0, "x mag"=0, "y mag"=0, "z mag"=0} ("Raw IMU"), "x acc"=w207, "y acc"=w208, "z acc"=w209, "x gyro"=w215, "y gyro"=w210, "z gyro"=w211, "x mag"=w212, "y mag"=w213, "z mag"=w214) -> ()  [unwired: 1 out]
            n75 = call "Disable Data Stream.vi"("error in (no error)"=w182, "req_stream_id"=T19."RAW_SENSORS", "Aircraft ID"=w180) -> ("error out"=w183:errorcluster)  [unwired: 8 in]
          }
          frame 30 {
            w242 = 4 ("length")
            # "Attitude"
            n76 = String To Byte Array(string=w229) -> (unsigned byte array=w241:u8[])
            n77 = Array Subset(array=w241, index=4, length=w242) -> (w232:u8[])
            n78 = Array Subset(array=w241, length=w242) -> (w243:u8[])  [unwired: 1 in]
            n79 = Array Subset(array=w241, index=8, length=w242) -> (w234:u8[])
            n80 = Array Subset(array=w241, index=12, length=w242) -> (w237:u8[])
            n81 = Reverse 1D Array(array=w243) -> (reversed array=w244:u8[])
            n82 = Reverse 1D Array(array=w232) -> (reversed array=w233:u8[])
            n83 = Reverse 1D Array(array=w234) -> (reversed array=w238:u8[])
            n84 = Reverse 1D Array(array=w237) -> (reversed array=w239:u8[])
            n85 = Type Cast(type=u32 0 ("single precision float"), x=w244) -> (*(type *) &x=w228:u32)
            n86 = Type Cast(type=sgl 0.0 ("single precision float"), x=w233) -> (*(type *) &x=w246:sgl)
            n87 = Type Cast(type=w246, x=w238) -> (*(type *) &x=w247:sgl)
            n88 = Type Cast(type=w247, x=w239) -> (*(type *) &x=w248:sgl)
            n89 = expression code="(x/pi)*180.0" "radians to degrees"(w247) -> (w252:sgl)
            n90 = expression code="(x/pi)*180.0" "radians to degrees"(w246) -> (w251:sgl)
            n91 = expression code="(x/pi)*180.0" "radians to degrees"(w248) -> (w249:sgl)
            n92 = call <vilib>:"High Resolution Relative Seconds.vi"() -> ("relative seconds"=w226:dbl)
            n93 = Sign(1:w249) -> (0:w240:sgl)
            n94 = case shown="-1" w240 {
              tunnel: w249 -> [w254 w256 w257]
              tunnel: [w253 w256 w257] -> w250
              frame -1 {
                n95 = Add(x=sgl 360.0, y=w254) -> (x+y=w253:sgl)
              }
              frame 0, Default {
              }
              frame 1 {
              }
            }
            n96 = feedback-in #1(w226) -> ()
            n97 = feedback #1() -> (w227:dbl)  [unwired: 1 in]
            n98 = Subtract(x=w226, y=w227) -> (x-y=w225:dbl)
            n99 = Reciprocal(x=w225) -> (1/x=w224:dbl)
            n100 = Bundle By Name(cluster=w221, "Timestamp"=w228, "Roll"=w251, "Pitch"=w252, "Yaw"=w250, "Update Frequency"=w224) -> (w220:T6)
          }
          frame 33 {
            w277 = sgl 10000000.0
            w276 = 4 ("length")
            # "GPS Position"
            n101 = String To Byte Array(string=w266) -> (unsigned byte array=w282:u8[])
            n102 = Array Subset(array=w282, index=4, length=w276) -> (w268:u8[])
            n103 = Array Subset(array=w282, index=8, length=w276) -> (w270:u8[])
            n104 = Array Subset(array=w282, index=12, length=w276) -> (w273:u8[])
            n105 = Array Subset(array=w282, index=26, length=2) -> (w287:u8[])
            n106 = Reverse 1D Array(array=w268) -> (reversed array=w269:u8[])
            n107 = Reverse 1D Array(array=w270) -> (reversed array=w274:u8[])
            n108 = Reverse 1D Array(array=w273) -> (reversed array=w275:u8[])
            n109 = Reverse 1D Array(array=w287) -> (reversed array=w288:u8[])
            n110 = Type Cast(type=u16 0, x=w288) -> (*(type *) &x=w285:u16)
            n111 = Type Cast(type=0, x=w269) -> (*(type *) &x=w278:i32)
            n112 = Type Cast(type=w278, x=w274) -> (*(type *) &x=w279:i32)
            n113 = Type Cast(type=w279, x=w275) -> (*(type *) &x=w280:i32)
            n114 = Divide(x=w285, y=u16 100) -> (x/y=w294:dbl)
            n115 = Divide(x=w278, y=w277) -> (x/y=w291:sgl)
            n116 = Divide(x=w279, y=w277) -> (x/y=w292:sgl)
            n117 = Divide(x=w280, y=sgl 1000.0) -> (x/y=w293:sgl)
            n118 = Bundle By Name(cluster=w263, "Latitude (degrees)"=w291, "Longitude (degrees)"=w292, "Altitude (m)"=w293, "Fix Type"=w294) -> (w262:T7)
          }
          frame 74 {
            # "VFR_HUD"
            n119 = String To Byte Array(string=w307) -> (unsigned byte array=w306:u8[])
            n120 = Array Subset(array=w306, index=8, length=4) -> (w309:u8[])
            n121 = Reverse 1D Array(array=w309) -> (reversed array=w310:u8[])
            n122 = Type Cast(type=sgl 0.0 ("single precision float"), x=w310) -> (*(type *) &x=w304:sgl)
            n123 = Bundle By Name(cluster=w300, "Altitude"=w304) -> (w299:T6)
          }
          frame 35 {
            w339 = 2 ("index")
            # "RC Channel IN"
            n124 = String To Byte Array(string=w320) -> (unsigned byte array=w338:u8[])
            n125 = Array Subset(array=w338, index=18, length=w339) -> (w334:u8[])
            n126 = Array Subset(array=w338, index=10, length=w339) -> (w323:u8[])
            n127 = Array Subset(array=w338, index=16, length=w339) -> (w336:u8[])
            n128 = Array Subset(array=w338, index=12, length=w339) -> (w330:u8[])
            n129 = Array Subset(array=w338, index=14, length=w339) -> (w333:u8[])
            n130 = Array Subset(array=w338, index=4, length=w339) -> (w328:u8[])
            n131 = Array Subset(array=w338, index=8, length=w339) -> (w322:u8[])
            n132 = Array Subset(array=w338, index=6, length=w339) -> (w329:u8[])
            n133 = Reverse 1D Array(array=w330) -> (reversed array=w344:u8[])
            n134 = Reverse 1D Array(array=w328) -> (reversed array=w340:u8[])
            n135 = Reverse 1D Array(array=w329) -> (reversed array=w341:u8[])
            n136 = Reverse 1D Array(array=w323) -> (reversed array=w343:u8[])
            n137 = Reverse 1D Array(array=w333) -> (reversed array=w345:u8[])
            n138 = Reverse 1D Array(array=w322) -> (reversed array=w342:u8[])
            n139 = Reverse 1D Array(array=w334) -> (reversed array=w347:u8[])
            n140 = Reverse 1D Array(array=w336) -> (reversed array=w346:u8[])
            n141 = Type Cast(type=u16 0, x=w340) -> (*(type *) &x=w349:u16)
            n142 = Type Cast(type=w349, x=w341) -> (*(type *) &x=w350:u16)
            n143 = Type Cast(type=w350, x=w342) -> (*(type *) &x=w351:u16)
            n144 = Type Cast(type=w351, x=w343) -> (*(type *) &x=w352:u16)
            n145 = Type Cast(type=w352, x=w344) -> (*(type *) &x=w353:u16)
            n146 = Type Cast(type=w353, x=w345) -> (*(type *) &x=w354:u16)
            n147 = Type Cast(type=w354, x=w346) -> (*(type *) &x=w355:u16)
            n148 = Type Cast(type=w355, x=w347) -> (*(type *) &x=w356:u16)
            n149 = Bundle By Name(cluster=T21 {"Channel 1"=0, "Channel 2"=0, "Channel 3"=0, "Channel 4"=0, "Channel 5"=0, "Channel 6"=0, "Channel 7"=0, "Channel 8"=0} ("RC CH IN"), "Channel 1"=w349, "Channel 2"=w350, "Channel 3"=w351, "Channel 4"=w352, "Channel 5"=w353, "Channel 6"=w354, "Channel 7"=w355, "Channel 8"=w356) -> ()  [unwired: 1 out]
            n150 = call "Disable Data Stream.vi"("error in (no error)"=w318, "req_stream_id"=T19."RC_CHANNELS", "Aircraft ID"=w316) -> ("error out"=w319:errorcluster)  [unwired: 8 in]
          }
          frame 36 {
            w393 = 2 ("index")
            # "RC Channel OUT"
            n151 = String To Byte Array(string=w375) -> (unsigned byte array=w394:u8[])
            n152 = Array Subset(array=w394, index=18, length=w393) -> (w389:u8[])
            n153 = Array Subset(array=w394, index=10, length=w393) -> (w378:u8[])
            n154 = Array Subset(array=w394, index=16, length=w393) -> (w391:u8[])
            n155 = Array Subset(array=w394, index=12, length=w393) -> (w385:u8[])
            n156 = Array Subset(array=w394, index=14, length=w393) -> (w388:u8[])
            n157 = Array Subset(array=w394, index=4, length=w393) -> (w383:u8[])
            n158 = Array Subset(array=w394, index=8, length=w393) -> (w377:u8[])
            n159 = Array Subset(array=w394, index=6, length=w393) -> (w384:u8[])
            n160 = Reverse 1D Array(array=w383) -> (reversed array=w395:u8[])
            n161 = Reverse 1D Array(array=w385) -> (reversed array=w399:u8[])
            n162 = Reverse 1D Array(array=w389) -> (reversed array=w402:u8[])
            n163 = Reverse 1D Array(array=w378) -> (reversed array=w398:u8[])
            n164 = Reverse 1D Array(array=w388) -> (reversed array=w400:u8[])
            n165 = Reverse 1D Array(array=w377) -> (reversed array=w397:u8[])
            n166 = Reverse 1D Array(array=w391) -> (reversed array=w401:u8[])
            n167 = Reverse 1D Array(array=w384) -> (reversed array=w396:u8[])
            n168 = Type Cast(type=u16 0, x=w395) -> (*(type *) &x=w373:u16)
            n169 = Type Cast(type=w373, x=w396) -> (*(type *) &x=w372:u16)
            n170 = Type Cast(type=w372, x=w397) -> (*(type *) &x=w371:u16)
            n171 = Type Cast(type=w371, x=w398) -> (*(type *) &x=w370:u16)
            n172 = Type Cast(type=w370, x=w399) -> (*(type *) &x=w369:u16)
            n173 = Type Cast(type=w369, x=w400) -> (*(type *) &x=w368:u16)
            n174 = Type Cast(type=w368, x=w401) -> (*(type *) &x=w367:u16)
            n175 = Type Cast(type=w367, x=w402) -> (*(type *) &x=w366:u16)
            n176 = Bundle By Name(cluster=T21 {"Channel 1"=0, "Channel 2"=0, "Channel 3"=0, "Channel 4"=0, "Channel 5"=0, "Channel 6"=0, "Channel 7"=0, "Channel 8"=0} ("RC CH OUT"), "Channel 1"=w373, "Channel 2"=w372, "Channel 3"=w371, "Channel 4"=w370, "Channel 5"=w369, "Channel 6"=w368, "Channel 7"=w367, "Channel 8"=w366) -> ()  [unwired: 1 out]
            n177 = call "Disable Data Stream.vi"("error in (no error)"=w363, "req_stream_id"=T19."RC_CHANNELS", "Aircraft ID"=w362) -> ("error out"=w364:errorcluster)  [unwired: 8 in]
          }
          frame 39, 40, 44, 47 {
            # "Queue up mission Items in Waypoint queue including:\nMission ACK, Mission Count, Mission Item, Mission Request"
            n178 = Lossy Enqueue Element(queue=w412, element=w411, error in (no error)=w410) -> (error out=w409:errorcluster)  [unwired: 3 out]
          }
          frame 77 {
            w427 = T1 {"Command ID"=0, "Command Result"=""}  # COMMAND ACK
            # "Command Acknowledge"
            n179 = String To Byte Array(string=w436) -> (unsigned byte array=w434:u8[])
            n180 = Array Subset(array=w434, length=2) -> (w438:u8[])  [unwired: 1 in]
            n181 = Array Subset(array=w434, index=2, length=1) -> (w431:u8[])
            n182 = Reverse 1D Array(array=w431) -> (reversed array=w429:u8[])
            n183 = Reverse 1D Array(array=w438) -> (reversed array=w437:u8[])
            n184 = Type Cast(type=u8 0, x=w429) -> (*(type *) &x=w428:u8)
            n185 = Type Cast(type=u16 0, x=w437) -> (*(type *) &x=w426:u16)
            n186 = case shown="4" w428 {
              tunnel: ["Command ACCEPTED and EXECUTED" "Command TEMPORARY REJECTED/DENIED" "Command PERMANENTLY DENIED" "Command UNKNOWN/UNSUPPORTED" "Command executed, but failed"] -> w424
              frame 0, Default {
              }
              frame 1 {
              }
              frame 2 {
              }
              frame 3 {
              }
              frame 4 {
              }
            }
            n187 = Unbundle By Name(w420) -> ("Status text"=w425:string)
            n188 = Concatenate Strings(w425, w424, "\n") -> (w422:string)
            n189 = Bundle By Name(cluster=w427, "Command ID"=w426, "Command Result"=w424) -> (→"output cluster":T1)
            n190 = Bundle By Name(cluster=w420, "Status text"=w422) -> (w418:T9)
          }
          frame 100 {
            # "Optical Flow Data"
            n191 = call "Parse OPTICAL_FLOW.vi"("Data"=w454) -> ("Optical Flow Data"=w453:T13)  [unwired: 10 in]
            n192 = Bundle By Name(cluster=w451, "Optical Flow"=w453) -> (w450:T12)
          }
          frame 173 {
            # "Rangfinder Data"
            n193 = call "Parse RANGEFINDER.vi"("Data"=w465) -> ("Voltage"=w463:sgl, "Distance (m)"=w464:sgl)  [unwired: 9 in]
            n194 = Bundle By Name(cluster=w461, "RNGFND Distance (m)"=w464, "RNGFND Voltage"=w463) -> (w460:T12)
          }
          frame 193 {
            # "EKF Status Report"
            n195 = call "Parse EKF_STATUS_REPORT.vi"("Data"=w475) -> ("EKF Status Report"=w474:T14)  [unwired: 10 in]
            n196 = Bundle By Name(cluster=w472, "EKF Status Report"=w474) -> (w470:T12)
          }
          frame 253 {
            w484 = 100  # Max Number of Messages to Display
            # "Status Text"
            n197 = String To Byte Array(string=w496) -> (unsigned byte array=w492:u8[])
            n198 = Array Subset(array=w492, index=1, length=50) -> (w489:u8[])
            n199 = Array Subset(array=w492, length=1) -> (w494:u8[])  [unwired: 1 in]
            n200 = Byte Array To String(unsigned byte array=w489) -> (string=w487:string)
            n201 = Type Cast(type=u8 0, x=w494) -> (*(type *) &x=w486:u8)
            n202 = Unbundle By Name(w482) -> ("Status text"=w488:string)
            n203 = call "Concatenate Status Text String.vi"("Max Number of Messages to Display"=w484, "Severity"=w486, "New Status Message"=w487, "Status Text"=w488) -> ("Output"=w485:string)  [unwired: 7 in]
            n204 = Bundle By Name(cluster=w482, "Status text"=w485) -> (w481:T9)
          }
          frame Default {
            # "unknown message"
          }
        }
      }
      frame True {
        # "Timed out. nothing received\nmark coms with aircraft as bad"
        n205 = Bundle By Name(cluster=w506, "Coms with aircraft good"=FALSE) -> (w505:T15)
      }
    }
    n206 = call-poly "Stop Button.vi"() -> ("Stop ButtonOut"=w28:bool)  [unwired: 10 in, 1 out]
    n207 = call-poly "Aircraft Info.vi"("Aircraft ID"=w14, "Aircraft Information In"=w22) -> ("Aircraft Information Out"=w23:T15)  [unwired: 8 in, 1 out]
    n208 = call-poly "Aircraft System Status.vi"("Aircraft ID"=w14, "System Status In"=w21) -> ("System Status Out"=w25:T9)  [unwired: 8 in, 1 out]
    n209 = call-poly "Aircraft Extra Data.vi"("Aircraft ID"=w14, "Extra Data In"=w18) -> ("Extra Data Out"=w19:T12)  [unwired: 8 in, 1 out]
    n210 = call-poly "Aircraft GPS.vi"("Aircraft ID"=w14, "Aircraft Att Data IN"=w15) -> ("Aircraft Att Data Out"=w17:T7)  [unwired: 8 in, 1 out]
    n211 = call-poly "Aircraft Attitude.vi"("Aircraft ID"=w14, "Aircraft Att Data In"=w11) -> ("Aircraft Att Data Out"=w13:T6)  [unwired: 8 in, 1 out]
    n212 = call "Error.vi"("Error In"=w27) -> ()  [unwired: 10 in, 1 out]
  }
